vi "U3 Stream Example LJ_swALL_OR_NONE.vi"() -> ()   [LabVIEW 2021]
panel:
  in  "Resolution Index":u8
  out "Waveform Chart":dbl[][](graph)
  out "# Skipped Scans":i32
  in  "Simulated Processing Delay [ms]":u32
  out "UD Backlog [%]":dbl format="%.2f"
  in  "Scan List":u8[](array[numeric])=[0, 1, 2, 3]
  out "Actual Scan Rate (Hz)":dbl=1000.0 format="%.3f"
  out "ms Per Loop":u32
  out "U3 Backlog [%]":dbl format="%.2f"
  out "Scans Retrieved Sec (measured)":dbl format="%.2f"
  out "# Scans Read":i32
  out "# of iterations":i32
  out "Data":dbl[][](array[numeric]) format="%.3f"
  in  "Scan Rate (Hz)":dbl=1000.0 format="%.3f"
  in  "Data File Extension":string="dat"
  out "Current Data File":path
  in  "Data File Prefix":string="data"
  in  "Write To File":bool
  in  "FirstFound":bool=TRUE
  in  "stop":bool
  in  "Address":string="1"
  out "Error Message":string
  # "Streams using the ALL_OR_NONE wait mode.  Streaming\nrequires U3 hardware revision 1.21."
  # "The actual scans/sec is controlled\nby hardware and is known.  This\n\"measured\" suggests the rate at\nwhich data is being retreived."
  # "0=Auto"
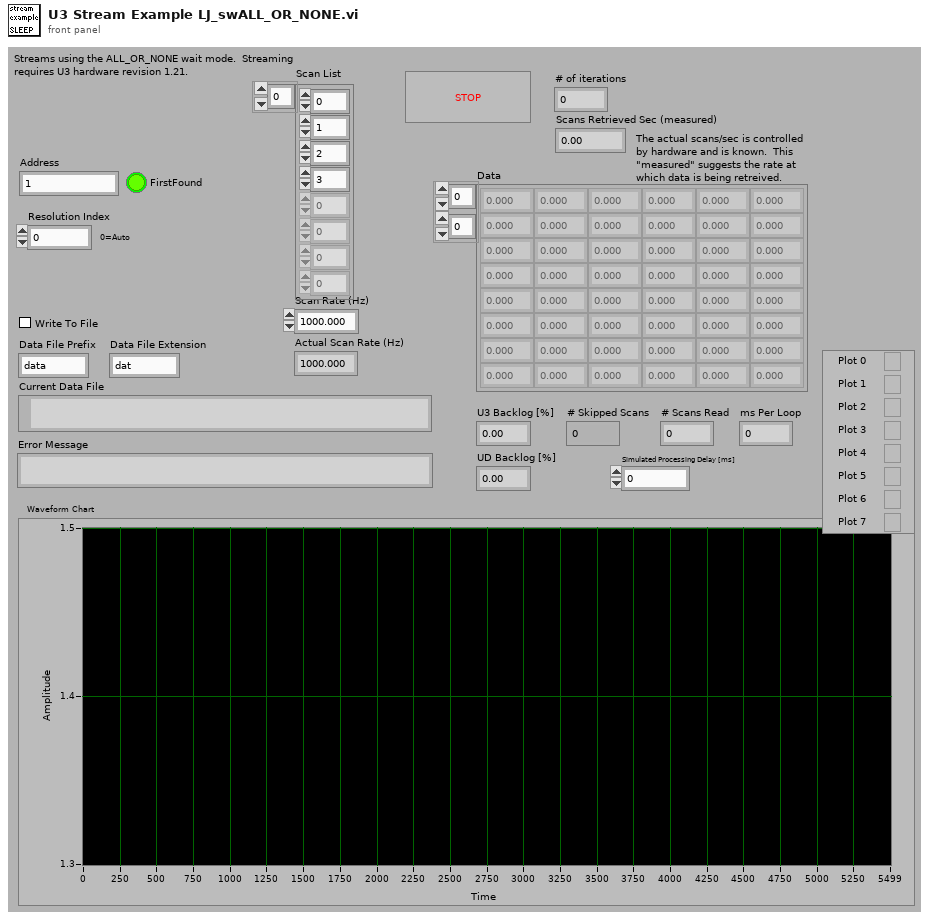
[diagram p1: front panel]
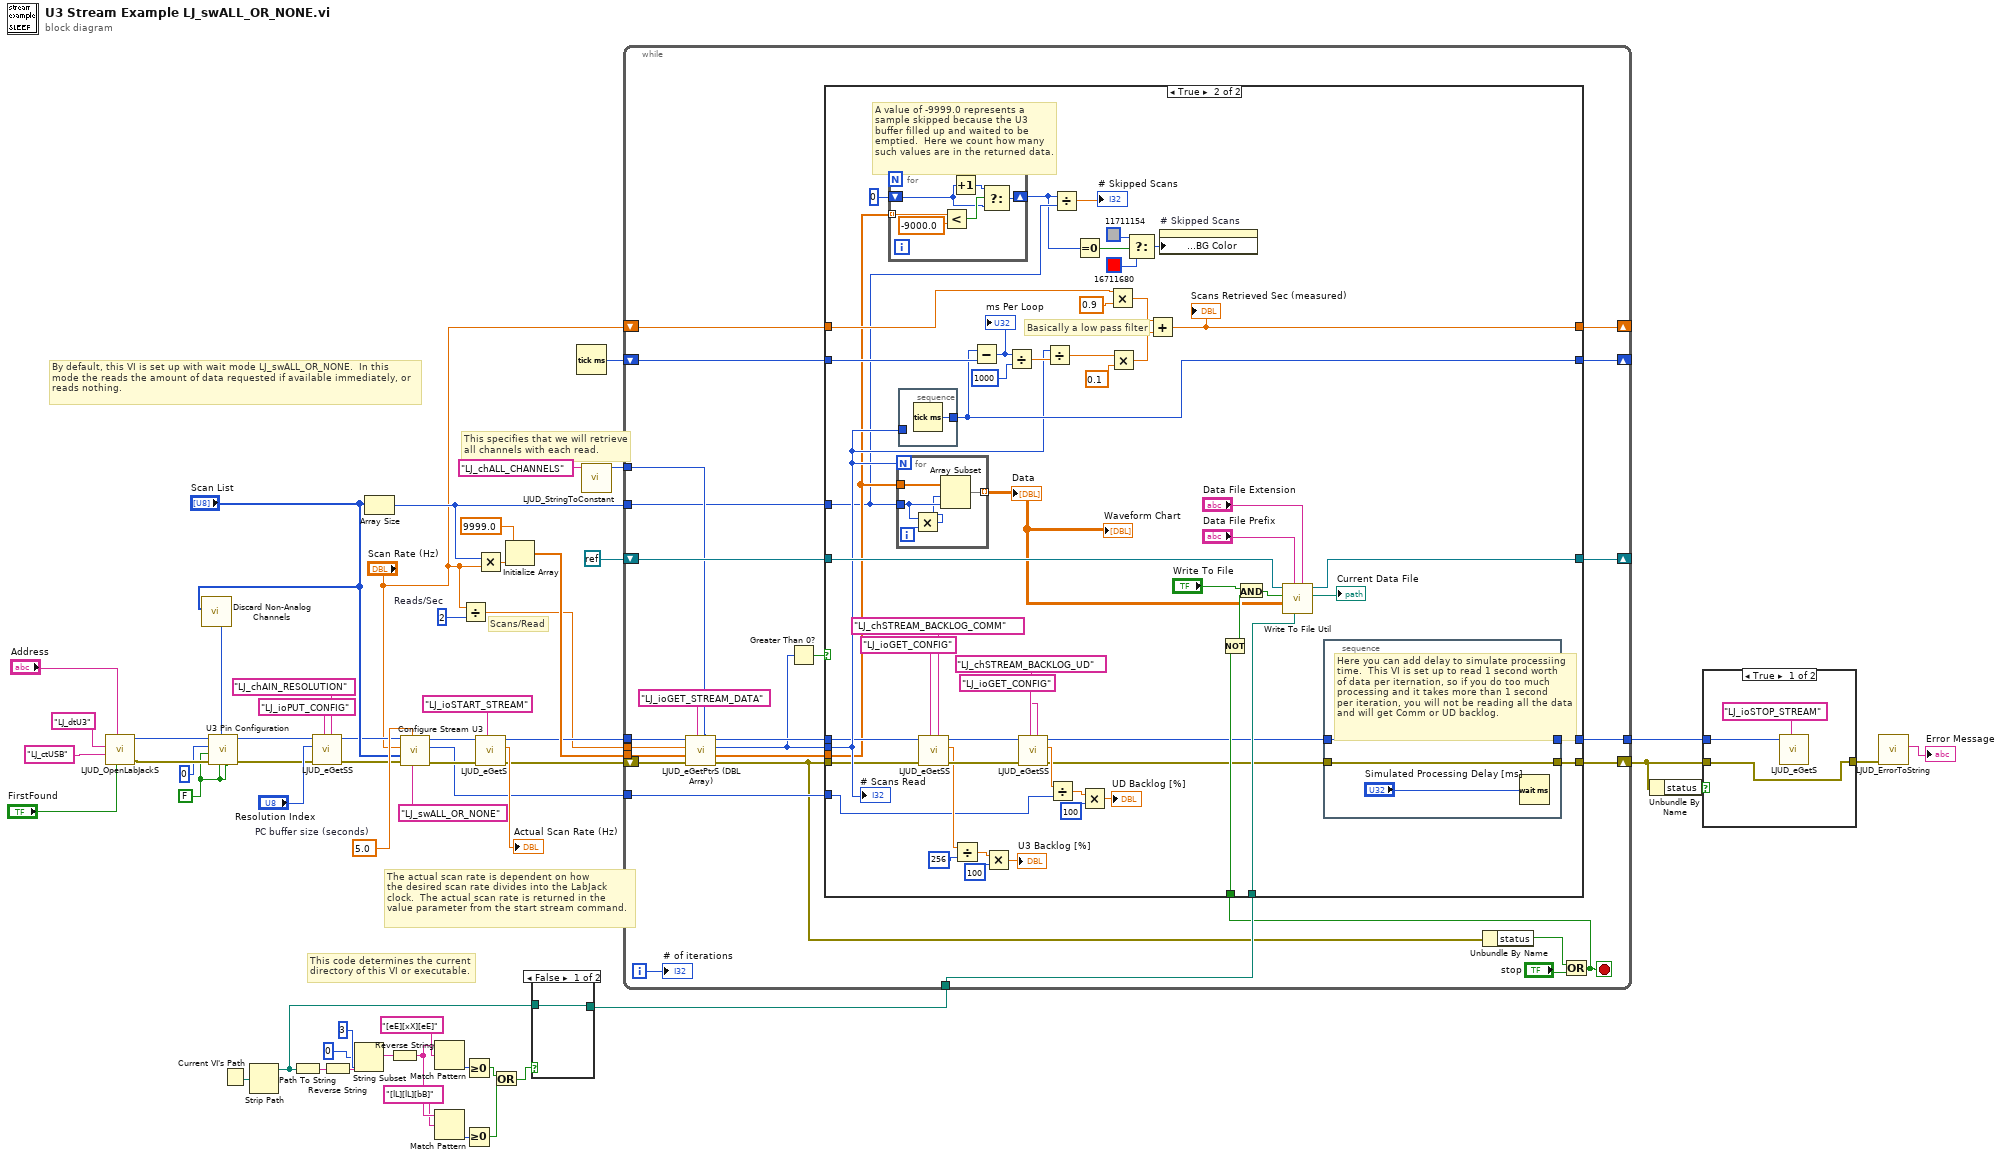
[diagram p0: block diagram]
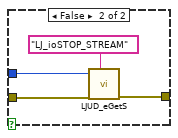
[diagram p3: hidden frame]
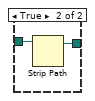
[diagram p4: hidden frame]
diagram:
  w3 = 2  # Reads/Sec
  w14 = FALSE ("Enable DAC1")
  w27 = 5.0  # PC buffer size (seconds)
  # "Scans/Read"
  # "This specifies that we will retrieve\nall channels with each read."
  # "The actual scan rate is dependent on how\nthe desired scan rate divides into the LabJack\nclock.  The actual scan rate is returned in the\nvalue parameter from the start stream command."
  # "By default, this VI is set up with wait mode LJ_swALL_OR_NONE.  In this\nmode the reads the amount of data requested if available immediately, or\nreads nothing."
  # "This code determines the current\ndirectory of this VI or executable."
  n1 = call "LJUD_OpenLabJackS.vi"("FirstFound"="FirstFound", "Address"="Address", "ConnectionType"="LJ_ctUSB", "DeviceType"="LJ_dtU3") -> ("error out"=w17:errorcluster, "Handle"=w18:i32)  [unwired: 5 in, 1 out]
  n2 = call "Discard Non-Analog Channels.vi"("Channels In"="Scan List") -> ("FIO/EIO Analog Enable"=w13:i32)  [unwired: 7 in, 3 out]
  n3 = call "U3 Pin Configuration.vi"("Enable Counter1"=w14, "Enable Counter0"=w14, "FIO/EIO Analog Enable"=w13, "error in"=w17, "Enable DAC1"=w14, "Number of Timers Enabled"=u8 0, "Handle In"=w18) -> ("error out"=w7:errorcluster, "Handle Out"=w8:i32)  [unwired: 3 in]
  n4 = Current VI's Path() -> (path=w55:path)
  n5 = Strip Path(path=w55) -> (stripped path=w47:path)  [unwired: 1 out]
  n6 = Path To String(path=w47) -> (string=w54:string)
  n7 = call "LJUD_eGetSS.vi"("Channel"="LJ_chAIN_RESOLUTION", "IOType"="LJ_ioPUT_CONFIG", "error in"=w7, "Value Write"="Resolution Index", "Handle In"=w8) -> ("error out"=w6:errorcluster, "Handle Out"=w5:i32)  [unwired: 4 in, 1 out]
  n8 = Reverse String(1:w54) -> (0:w53:string)
  n9 = String Subset(string=w53, offset (0)=0, length (rest)=3 ("length")) -> (substring=w50:string)
  n10 = Array Size(array="Scan List") -> (size(s)=w33:i32)
  n11 = Reverse String(1:w50) -> (0:w46:string)
  n12 = call "Configure Stream U3.vi"("Wait Mode"="LJ_swALL_OR_NONE" ("Wait Mode (2)"), "PC buffer size (seconds)"=w27, "error in"=w6, "Scan List (+)"="Scan List", "Scan Rate (Hz)"="Scan Rate (Hz)", "Handle In"=w5) -> ("error out"=w37:errorcluster, "PC buffer size (samples)"=w19:i32, "Handle Out"=w38:i32)  [unwired: 3 in]
  n13 = Match Pattern(string=w46, regular expression="[eE][xX][eE]") -> (offset past match=w48:i32)  [unwired: 1 in, 3 out]
  n14 = Match Pattern(string=w46, regular expression="[lL][lL][bB]") -> (offset past match=w43:i32)  [unwired: 1 in, 3 out]
  n15 = Divide(x="Scan Rate (Hz)", y=w3) -> (x/y=w2:dbl)
  n16 = Greater Or Equal To 0?(x=w48) -> (x >= 0?=w44:bool)
  n17 = Greater Or Equal To 0?(x=w43) -> (x >= 0?=w42:bool)
  n18 = Multiply(x=w33, y="Scan Rate (Hz)") -> (x*y=w36:dbl)
  n19 = call "LJUD_eGetS.vi"("IOType"="LJ_ioSTART_STREAM", "error in"=w37, "Handle In"=w38) -> ("error out"=w21:errorcluster, "Value Read"=→"Actual Scan Rate (Hz)":dbl, "Handle Out"=w25:i32)  [unwired: 6 in]
  n20 = Or(x=w44, y=w42) -> (x .or. y?=w41:bool)
  n21 = Initialize Array(9999.0, w36) -> (w34:dbl[])
  n22 = case shown="False" w41 {
    tunnel: w47 -> [w59 w61]
    tunnel: [w59 w60] -> w40
    frame False {
    }
    frame True {
      n23 = Strip Path(path=w61) -> (stripped path=w60:path)  [unwired: 1 out]
    }
  }
  n24 = Tick Count (ms)() -> (millisecond timer value=w28:u32)
  n25 = call "LJUD_StringToConstant.vi"("String"="LJ_chALL_CHANNELS") -> ("Constant Number"=w22:i32)  [unwired: 9 in, 1 out]
  n26 = while {
    tunnel: w19 -> [w70]
    shift-left: w21 -> [w71]
    shift-right: [w65] -> w20
    tunnel: w22 -> [w72]
    shift-left: "Scan Rate (Hz)" -> [w75]
    shift-right: [w74] -> _
    shift-left: w28 -> [w77]
    shift-right: [w76] -> _
    tunnel: [w69] -> w31
    tunnel: w33 -> [w67]
    tunnel: w34 -> [w80]
    tunnel: w2 -> [w79]
    tunnel: w40 -> [w83]
    shift-left: refnum<k0> refnum -> [w85]
    shift-right: [w84] -> _
    tunnel: w25 -> [w82]
    i -> [w78]
    stop <- w66 stop-if-true
    n27 = call "LJUD_eGetPtrS (DBL Array).vi"("Channel"=w72, "IOType"="LJ_ioGET_STREAM_DATA", "error in"=w71, "DBL Array Write"=w80, "Value"=w79, "Handle In"=w82) -> ("error out"=w64:errorcluster, "DBL Array Read"=w68:dbl[], "Value"=w62:i32, "Handle Out"=w73:i32)  [unwired: 2 in]
    n28 = Greater Than 0?(x=w62) -> (x > 0?=w63:bool)
    n29 = Unbundle By Name(w64) -> ("status"=w86:bool)
    n30 = Or(x=w86, y="stop") -> (x .or. y?=w66:bool)
    n31 = case shown="True" w63 {
      tunnel: w85 -> [w90 w145]
      tunnel: [w90 w144] -> w84
      tunnel: w83 -> [_ w139]
      tunnel: w66 -> [_ w138]
      tunnel: w77 -> [w91 w137]
      tunnel: [w91 w134] -> w76
      tunnel: w62 -> [_ w132]
      tunnel: w75 -> [w92 w128]
      tunnel: [w92 w125] -> w74
      tunnel: w73 -> [w89 w124]
      tunnel: w64 -> [w88 w123]
      tunnel: w70 -> [_ w109]
      tunnel: [w88 w106] -> w65
      tunnel: [w89 w104] -> w69
      tunnel: w68 -> [_ w103]
      tunnel: w67 -> [_ w101]
      frame False {
      }
      frame True {
        # "A value of -9999.0 represents a\nsample skipped because the U3\nbuffer filled up and waited to be\nemptied.  Here we count how many\nsuch values are in the returned data."
        # "Basically a low pass filter"
        n32 = for {
          shift-right: [w148] -> w97
          shift-left: 0 -> [w149]
          tunnel: w103 -> [w152] mode=indexing
          n33 = Less?(x=w152, y=-9000.0) -> (x < y?=w150:bool)
          n34 = Increment(x=w149) -> (x+1=w153:i32)
          n35 = Select(t=w153, s=w150, f=w149) -> (s? t:f=w148:i32)
        }
        n36 = for {
          N: w132 -> [_]
          tunnel: w103 -> [w162]
          tunnel: w101 -> [w161]
          tunnel: [w158] -> w93 mode=indexing
          i -> [w160]
          n37 = Multiply(x=w161, y=w160) -> (x*y=w159:i32)
          n38 = Array Subset(array=w162, index=w159, length=w161) -> (w158:dbl[])
        }
        "Data" <- w93
        "Waveform Chart" <- w93
        n39 = stacked-sequence {
          tunnel: w132 -> [_]
          tunnel: [w157] -> w134
          frame #0 {
            n40 = Tick Count (ms)() -> (millisecond timer value=w157:u32)
          }
        }
        n41 = call "LJUD_eGetSS.vi"("Channel"="LJ_chSTREAM_BACKLOG_COMM", "IOType"="LJ_ioGET_CONFIG", "error in"=w123, "Handle In"=w124) -> ("error out"=w117:errorcluster, "Value Read"=w113:dbl, "Handle Out"=w118:i32)  [unwired: 5 in]
        n42 = Divide(x=w113, y=256) -> (x/y=w116:dbl)
        n43 = Subtract(x=w134, y=w137) -> (x-y=w136:u32)
        "ms Per Loop" <- w136
        n44 = Multiply(x=w116, y=100) -> (x*y=→"U3 Backlog [%]":dbl)
        n45 = Divide(x=w136, y=u32 1000) -> (x/y=w133:dbl)
        n46 = call "LJUD_eGetSS.vi"("Channel"="LJ_chSTREAM_BACKLOG_UD", "IOType"="LJ_ioGET_CONFIG", "error in"=w117, "Handle In"=w118) -> ("error out"=w94:errorcluster, "Value Read"=w108:dbl, "Handle Out"=w105:i32)  [unwired: 5 in]
        n47 = Divide(x=w132, y=w133) -> (x/y=w131:dbl)
        n48 = Divide(x=w108, y=w109) -> (x/y=w110:dbl)
        n49 = Divide(x=w97, y=w101) -> (x/y=→"# Skipped Scans":dbl)
        n50 = Equal To 0?(x=w97) -> (x = 0?=w96:bool)
        n51 = Multiply(x=w110, y=100) -> (x*y=→"UD Backlog [%]":dbl)
        n52 = Multiply(x=w128, y=0.9) -> (x*y=w127:dbl)
        n53 = Multiply(x=w131, y=0.1) -> (x*y=w126:dbl)
        n54 = Select(t=u32 11711154, s=w96, f=u32 16711680) -> (s? t:f=w95:u32)
        n55 = Add(x=w127, y=w126) -> (x+y=w125:dbl)
        "Scans Retrieved Sec (measured)" <- w125
        n56 = property on="# Skipped Scans" class="DigNum (strict)"("Numeric Text.Text Colors:BG Color"=w95) -> ()  [unwired: 2 in, 2 out]
        n57 = Not(x=w138) -> (.not. x?=w140:bool)
        n58 = And(x="Write To File", y=w140) -> (x .and. y?=w141:bool)
        n59 = call "Write To File Util.vi"("Data File Extension"="Data File Extension", "Working Directory"=w139, "Data File Prefix"="Data File Prefix", "Data"=w93, "Write To File"=w141, "File Refnum In"=w145) -> ("Current Data File"=→"Current Data File":path, "File Refnum Out"=w144:refnum<file>)  [unwired: 3 in, 1 out]
        n60 = stacked-sequence {
          tunnel: w94 -> [w156]
          tunnel: [w156] -> w106
          tunnel: w105 -> [w155]
          tunnel: [w155] -> w104
          frame #0 {
            # "Here you can add delay to simulate processiing\ntime.  This VI is set up to read 1 second worth\nof data per iternation, so if you do too much\nprocessing and it takes more than 1 second\nper iteration, you will not be reading all the data\nand will get Comm or UD backlog."
            n61 = Wait (ms)(milliseconds to wait="Simulated Processing Delay [ms]") -> ()  [unwired: 1 out]
          }
        }
        "# Scans Read" <- w132
      }
    }
    "# of iterations" <- w78
  }
  n62 = Unbundle By Name(w20) -> ("status"=w24:bool)
  n63 = case shown="True" w24 {
    tunnel: w31 -> [w164 w168]
    tunnel: [w163 w167] -> w30
    tunnel: w20 -> [w163 w166]
    frame True {
      n64 = call "LJUD_eGetS.vi"("IOType"="LJ_ioSTOP_STREAM", "Handle In"=w164) -> ()  [unwired: 7 in, 3 out]
    }
    frame False {
      n65 = call "LJUD_eGetS.vi"("IOType"="LJ_ioSTOP_STREAM", "error in"=w166, "Handle In"=w168) -> ("error out"=w167:errorcluster)  [unwired: 6 in, 2 out]
    }
  }
  n66 = call "LJUD_ErrorToString.vi"("error in"=w30) -> ("String"=→"Error Message":string)  [unwired: 10 in]
